vi "Read Step.vi"(8 "error in (no error)":errorcluster, 11 "Fortress In":refnum<class "Fortress.lvclass">) -> (0 "error out":errorcluster, 2 "Step":i32, 3 "Fortress Out":refnum<class "Fortress.lvclass">)   [LabVIEW 2015, in "Fortress.lvclass"]
uses:
  Fortress.lvclass
  Fortress.lvclass/Fortress.ctl
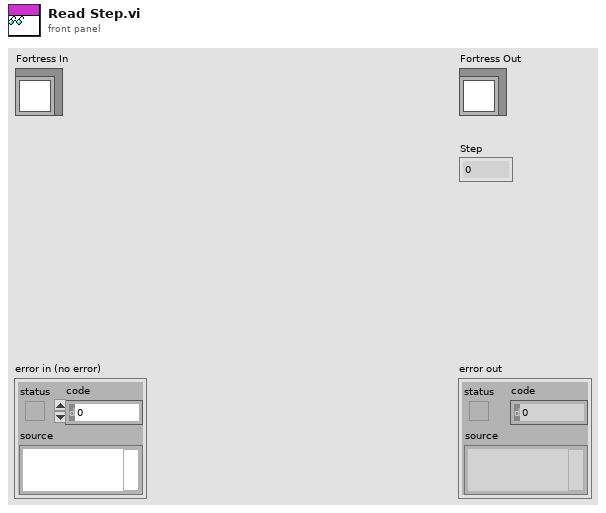
[diagram p1: front panel]
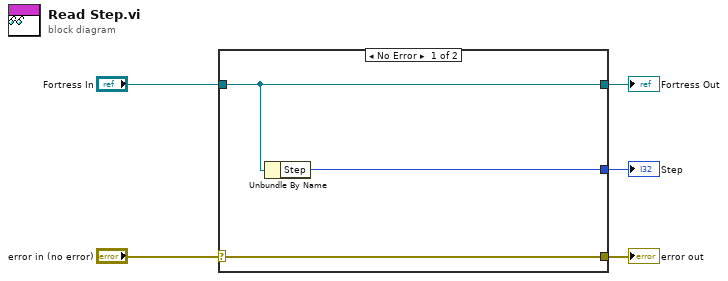
[diagram p0: block diagram]
diagram:
  n1 = case shown="No Error" "error in (no error)" {
    selector: "error in (no error)" -> [w8 w9]
    tunnel: [w8 w9] -> w4
    tunnel: [w7 w10] -> w2
    tunnel: "Fortress In" -> [w7 w10]
    tunnel: [w6 _] -> w1
    frame No Error {
      n2 = Unbundle By Name(w7) -> ("Step"=w6:i32)
    }
    frame Error {
    }
  }
  "error out" <- w4
  "Fortress Out" <- w2
  "Step" <- w1
